vi "DataTranslation.vi"() -> ()   [LabVIEW 2013]
doc: "This vi will take data with multiple DT boxes for an arbitrary number of channels either differentially or single ended, depending upon how you have wired the boxes up."
uses:
  Controls/DT_Cluster.ctl
  Controls/DT_Mode.ctl
  Globals/Meas_global.vi
  <userlib>/LV-Link3/PolySubVIs/DtCreateAinChan.vi
  <userlib>/LV-Link3/PolySubVIs/DtCreateCtrRateChan.vi
  <userlib>/LV-Link3/PolySubVIs/DtOLTimingSetInput.vi
  <userlib>/LV-Link3/PolySubVIs/DtOLStartNormal.vi
  <userlib>/LV-Link3/PolySubVIs/DtOLTriggerDigital.vi
  <userlib>/LV-Link3/PolySubVIs/DtOLReadMultiple2D.vi
panel:
  out "DAQ Error":errorcluster
  out "Array":T1[](array[typedef])
  out "Waveform Graph":dbl[][](graph)
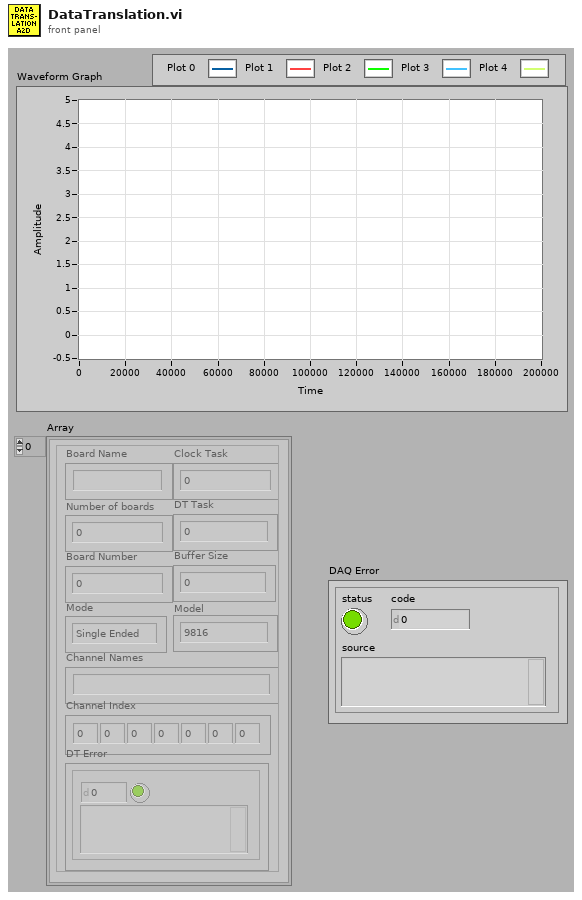
[diagram p1: front panel]
types:
  T1 = typedef "DT_Cluster.ctl" = cluster{"Board Name":string, "Number of boards":u32, "Board Number":u32, "Channel Names":string, "Channel Index":i32[], "DT Task":i32, "DT Error":errorcluster, "Mode":T2, "Buffer Size":u32, "Clock Task":i32, "Model":enum16{"9816", "9836", "9853"}}
  T2 = typedef "DT_Mode.ctl" = enum16{"Single Ended", "Differential"}
  T3 = typedef "Trigger_Mode.ctl" = enum16{"Free Running", "Start on Trigger", "Trigger Every Block", "Trigger Every Sample"}
  T4 = typedef "LDA_Setup.ctl" = cluster{"dimensions":enum16{"1D", "2D"}, "Analogue Freq Multiplier":dbl}
  T5 = enum32{"Internal Clock", "External Clock", "No Timing"}
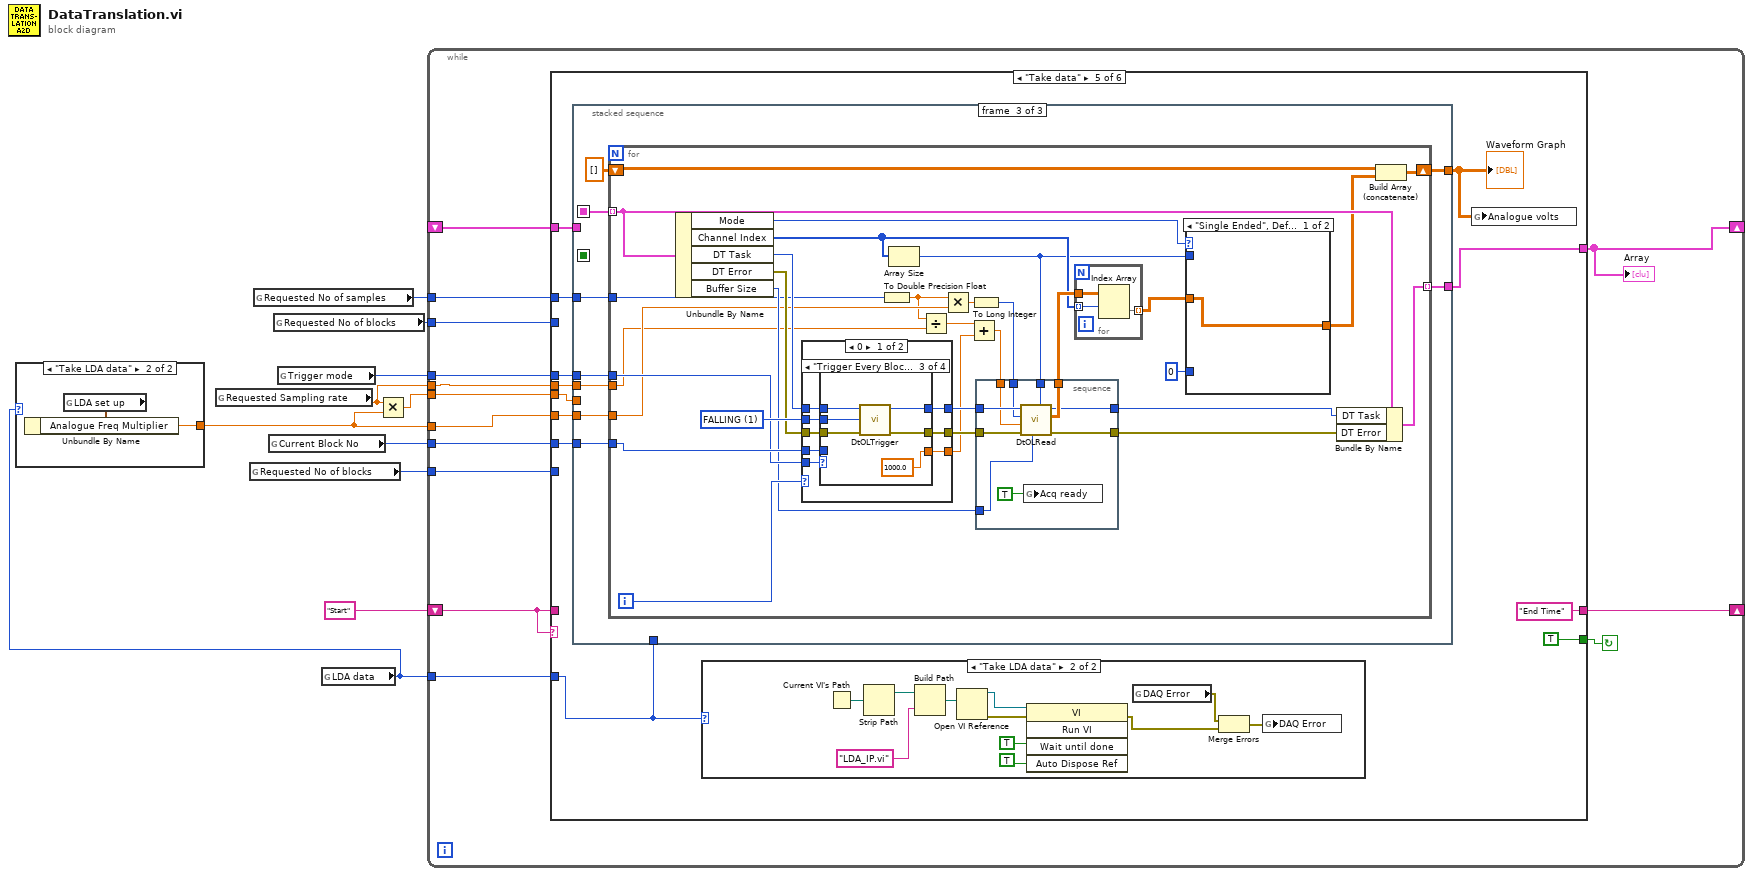
[diagram p0: block diagram]
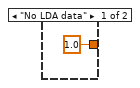
[diagram p2: hidden frame]
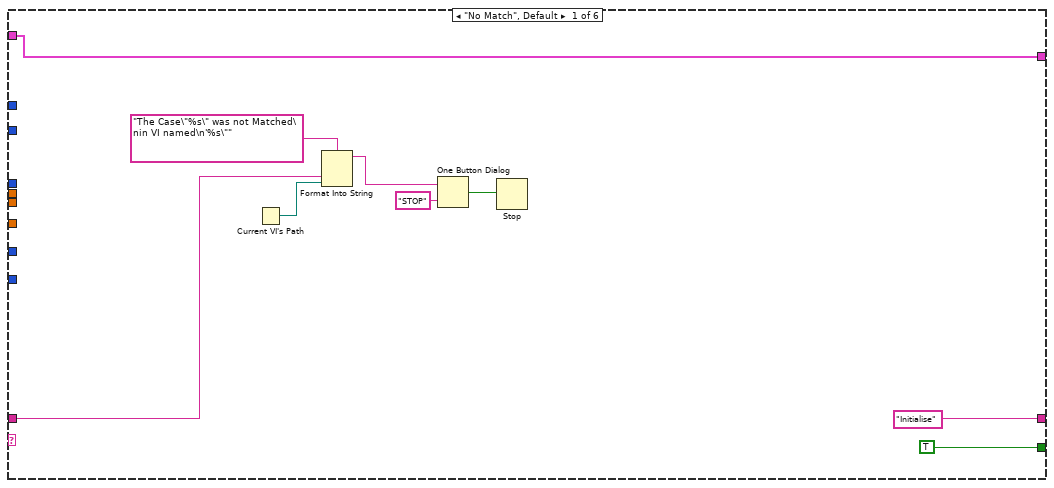
[diagram p3: hidden frame]
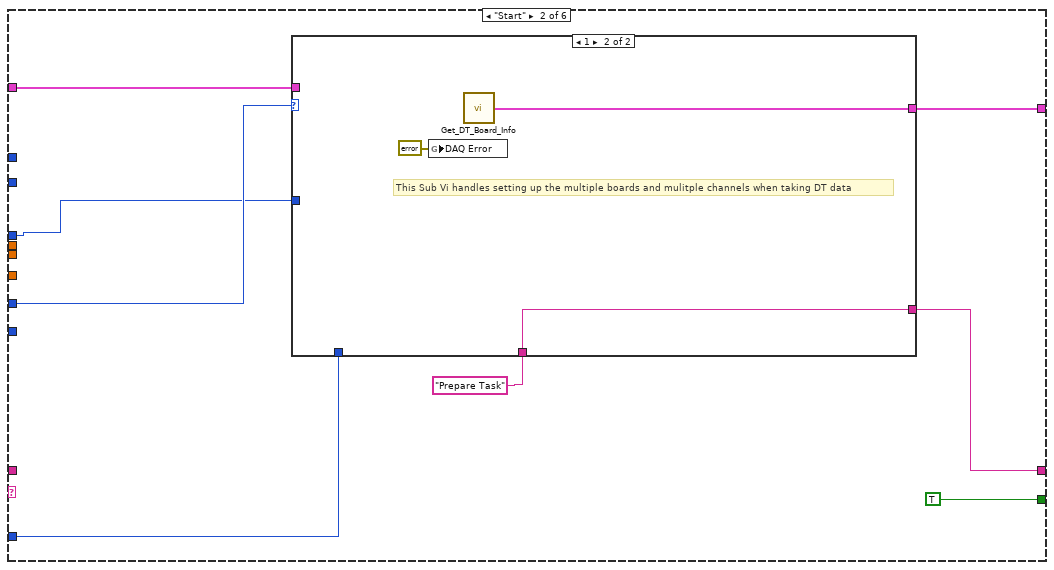
[diagram p4: hidden frame]
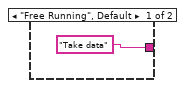
[diagram p6: hidden frame]
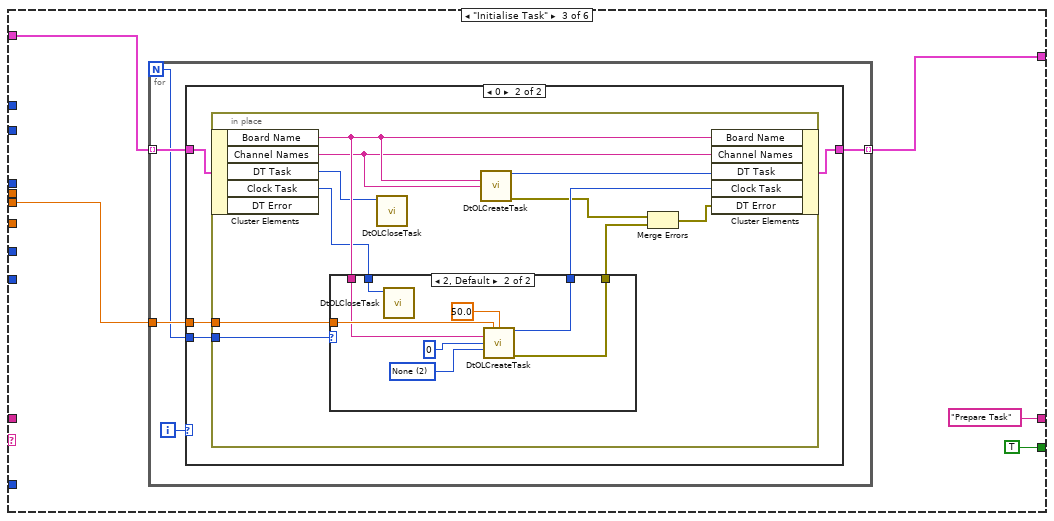
[diagram p8: hidden frame]
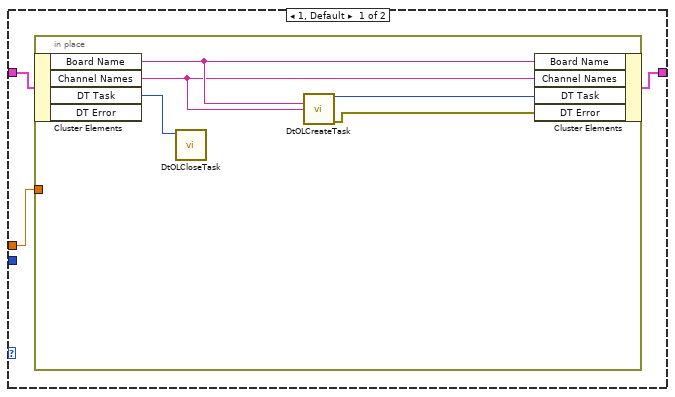
[diagram p9: hidden frame]
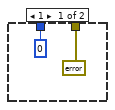
[diagram p10: hidden frame]
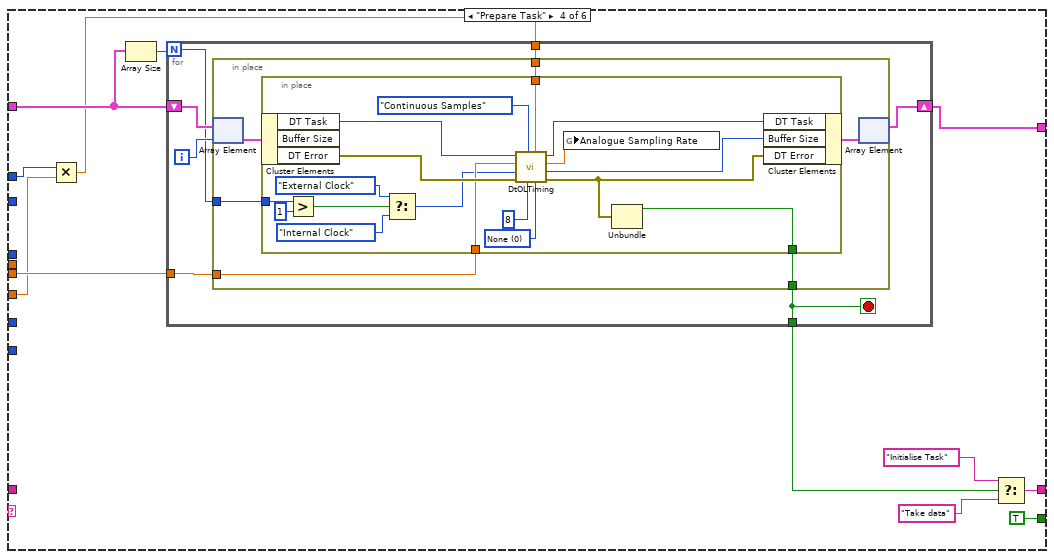
[diagram p11: hidden frame]
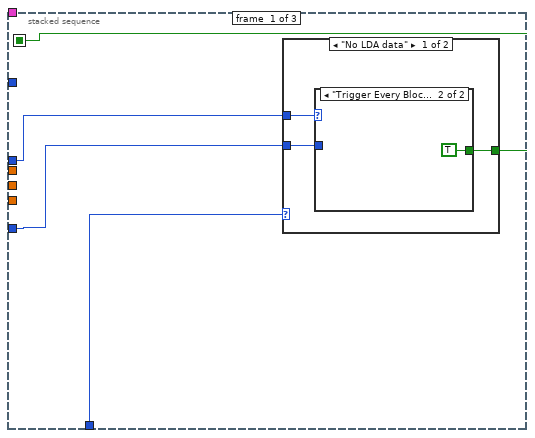
[diagram p13: hidden frame]
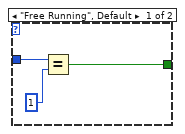
[diagram p14: hidden frame]
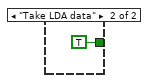
[diagram p15: hidden frame]
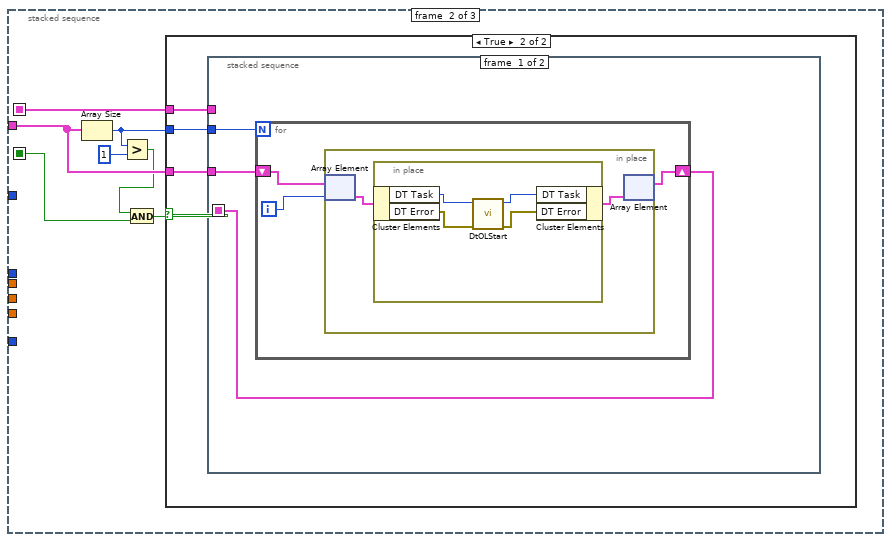
[diagram p16: hidden frame]
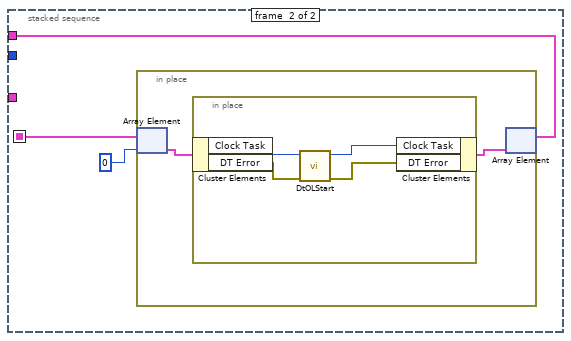
[diagram p18: hidden frame]
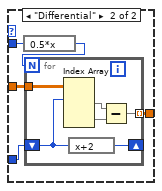
[diagram p19: hidden frame]
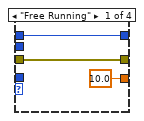
[diagram p20: hidden frame]
diagram:
  n1 = global read "Meas_global.vi" "Requested Sampling rate"() -> (w4:dbl)
  n2 = global read "Meas_global.vi" "Requested No of blocks"() -> (w3:i32)
  n3 = global read "Meas_global.vi" "Requested No of samples"() -> (w9:i32)
  n4 = global read "Meas_global.vi" "Current Block No"() -> (w7:i32)
  n5 = global read "Meas_global.vi" "Requested No of blocks"() -> (w6:i32)
  n6 = global read "Meas_global.vi" "Trigger mode"() -> (w8:T3)
  n7 = global read "Meas_global.vi" "LDA data"() -> (w1:enum16{"No LDA data", "Take LDA data"})
  n8 = case shown="\"Take LDA data\"" w1 {
    tunnel: [1.0 ("Analogue Freq Multiplier") w12] -> w2
    frame "No LDA data" {
    }
    frame "Take LDA data" {
      n9 = global read "Meas_global.vi" "LDA set up"() -> (w13:T4)
      n10 = Unbundle By Name(w13) -> ("Analogue Freq Multiplier"=w12:dbl)
    }
  }
  n11 = Multiply(x=w4, y=w2) -> (x*y=w5:dbl)
  n12 = while {
    shift-left: "Start" -> [w26]
    shift-right: [w27] -> _
    tunnel: w5 -> [w25]
    tunnel: w9 -> [w24]
    tunnel: w7 -> [w23]
    tunnel: w8 -> [w21]
    tunnel: w6 -> [w20]
    shift-right: [w19] -> _
    shift-left: _ -> [w18]
    tunnel: w1 -> [w17]
    tunnel: w2 -> [w16]
    tunnel: w4 -> [w15]
    tunnel: w3 -> [w14]
    stop <- w22 continue-if-true
    n13 = case shown="\"Take data\"" w26 {
      tunnel: ["Initialise" w40 "Prepare Task" w110 "End Time" "" ("f")] -> w27
      tunnel: w26 -> [w32 _ _ _ _ _]
      tunnel: w25 -> [_ _ w61 w106 w145 _]
      tunnel: w24 -> [_ _ _ w104 w155 _]
      tunnel: w23 -> [_ w41 _ _ w153 w319]
      tunnel: [TRUE TRUE TRUE TRUE TRUE FALSE] -> w22
      tunnel: w21 -> [_ w37 _ _ w152 _]
      tunnel: w20 -> [_ _ _ _ _ _]
      tunnel: w18 -> [w28 w42 w59 w105 w151 w323]
      tunnel: [w28 w43 w60 w107 w150 w322] -> w19
      tunnel: w17 -> [_ w38 _ _ w146 _]
      tunnel: w16 -> [_ _ _ w103 w148 _]
      tunnel: w15 -> [_ _ _ _ w147 _]
      tunnel: w14 -> [_ _ _ _ _ w320]
      frame "No Match", Default {
        n14 = Current VI's Path() -> (path=w31:path)
        n15 = Format Into String(format string="The Case\"%s\" was not Matched\nin VI named\n'%s\"" ("Format String"), w32, w31) -> (resulting string=w35:string)  [unwired: 2 in, 1 out]
        n16 = One Button Dialog(message=w35, button name ("OK")="STOP") -> (true=w33:bool)
        n17 = Stop(stop? (T)=w33) -> ()
      }
      frame "Start" {
        n18 = case shown="1" w41 {
          tunnel: [w49 w58] -> w43
          tunnel: w42 -> [w49 _]
          tunnel: [w47 w56] -> w40
          tunnel: "Prepare Task" -> [w46 w56]
          tunnel: w38 -> [w48 _]
          tunnel: w37 -> [w45 _]
          frame 2, Default {
            n19 = case shown="\"No LDA data\"" w48 {
              tunnel: [w52 w55] -> w47
              tunnel: w46 -> [w50 w55]
              tunnel: w45 -> [w51 _]
              frame "No LDA data" {
                n20 = case shown="\"Trigger Every Block\"" w51 {
                  tunnel: ["Take data" w54] -> w52
                  tunnel: w50 -> [_ w54]
                  frame "Free Running", Default {
                  }
                  frame "Trigger Every Block" {
                  }
                }
              }
              frame "Take LDA data" {
              }
            }
          }
          frame 1 {
            # "This Sub Vi handles setting up the multiple boards and mulitple channels when taking DT data"
            n21 = global write "Meas_global.vi" "DAQ Error"(errorcluster {"status"=FALSE, "code"=0, "source"=""} ("DAQ Error")) -> ()
            n22 = call "Get_DT_Board_Info.vi"() -> ("DT Cluster Array"=w58:T1[])  [unwired: 5 in]
          }
        }
      }
      frame "Initialise Task" {
        n23 = for {
          N -> [w64]
          tunnel: w59 -> [w68] mode=indexing
          tunnel: w61 -> [w67]
          tunnel: [w66] -> w60 mode=indexing
          i -> [w65]
          n24 = case shown="0" w65 {
            tunnel: w68 -> [w71 w80]
            tunnel: w67 -> [w70 w79]
            tunnel: [w69 w78] -> w66
            tunnel: w64 -> [_ w77]
            frame 1, Default {
              n25 = in-place {
                in-place-border: w70 -> [_]
                n26 = in-place-cluster #1(w71) -> ("Board Name"=w76:string, "Channel Names"=w73:string, "DT Task"=w72:i32)  [unwired: 1 out]
                n27 = call <userlib>:"DtOLCloseTask.vi"("Task in"=w72) -> ()  [unwired: 10 in, 1 out]
                n28 = call-poly <userlib>:"DtOLCreateTask.vi"("Board Name"=w76, "Channel"=w73) -> ("Task out"=w75:i32, "error out"=w74:errorcluster)  [unwired: 11 in, 1 out]
                n29 = in-place-cluster #1("Board Name"=w76, "Channel Names"=w73, "DT Task"=w75, "DT Error"=w74) -> (w69:T1)
              }
            }
            frame 0 {
              n30 = in-place {
                in-place-border: w79 -> [w91]
                in-place-border: w77 -> [w82]
                n31 = in-place-cluster #2(w80) -> ("Board Name"=w89:string, "Channel Names"=w84:string, "DT Task"=w83:i32, "Clock Task"=w81:i32)  [unwired: 1 out]
                n32 = case shown="2, Default" w82 {
                  tunnel: w91 -> [_ w98]
                  tunnel: [errorcluster {"status"=FALSE, "code"=0, "source"=""} ("error out") w97] -> w90
                  tunnel: w89 -> [_ w96]
                  tunnel: [0 ("Task out") w95] -> w87
                  tunnel: w81 -> [_ w94]
                  frame 1 {
                  }
                  frame 2, Default {
                    w101 = 2 items=["LowLevel", "HighLevel", "None"] ("Gate Type")
                    n33 = call <userlib>:"DtOLCloseTask.vi"("Task in"=w94) -> ()  [unwired: 10 in, 1 out]
                    n34 = call-poly <userlib>:"DtOLCreateTask.vi"("Requested\nFrequency (Hz)"=w98, "Duty Cycle"=50.0, "Board Name"=w96, "Counter Num"=u32 0, "Gate Type"=w101) -> ("Task out"=w95:i32, "error out"=w97:errorcluster)  [unwired: 8 in, 1 out]
                  }
                }
                n35 = call <userlib>:"DtOLCloseTask.vi"("Task in"=w83) -> ()  [unwired: 10 in, 1 out]
                n36 = call-poly <userlib>:"DtOLCreateTask.vi"("Board Name"=w89, "Channel"=w84) -> ("Task out"=w88:i32, "error out"=w86:errorcluster)  [unwired: 11 in, 1 out]
                n37 = Merge Errors(w86, w90) -> (w85:errorcluster)
                n38 = in-place-cluster #2("Board Name"=w89, "Channel Names"=w84, "DT Task"=w88, "Clock Task"=w87, "DT Error"=w85) -> (w78:T1)
              }
            }
          }
        }
      }
      frame "Prepare Task" {
        n39 = Multiply(x=w104, y=w103) -> (x*y=w102:dbl)
        n40 = Array Size(array=w105) -> (size(s)=w109:i32)
        n41 = for {
          N: w109 -> [w114]
          shift-right: [w117] -> w107
          shift-left: w105 -> [w119]
          tunnel: [w120] -> w108
          tunnel: w106 -> [w116]
          tunnel: w102 -> [w115]
          i -> [w118]
          stop <- w120 stop-if-true
          n42 = in-place {
            in-place-border: [w126] -> w120
            in-place-border: w116 -> [w123]
            in-place-border: w115 -> [w122]
            in-place-border: w114 -> [w121]
            n43 = in-place-array #3(w119, w118) -> (w125:T1)
            n44 = in-place {
              in-place-border: [w138] -> w126
              in-place-border: w123 -> [w137]
              in-place-border: w122 -> [w136]
              in-place-border: w121 -> [w135]
              w128 = 0 items=["None", "Master", "Slave"] ("Sync Mode")
              n45 = in-place-cluster #4(w125) -> ("DT Task"=w143:i32, "DT Error"=w142:errorcluster)  [unwired: 1 out]
              n46 = Greater?(x=w135, y=1) -> (0:w133:bool)
              n47 = Select(t=T5."External Clock" ("Timing"), s=w133, f=T5."Internal Clock" ("Timing")) -> (s? t:f=w130:T5)
              n48 = call-poly <userlib>:"DtOLTiming.vi"("Sync Mode"=w128, "Samples Per Channel"=w136, "Num Buffers"=u32 8, "Sample Mode"=enum16{"Finite Samples", "Continuous Samples"}."Continuous Samples", "error in (no error)"=w142, "Timing"=w130, "Sample Freq (Hz)"=w137, "Task in"=w143) -> ("error out"=w139:errorcluster, "Buffer Size"=w141:u32, "Actual Sample Freq"=w144:dbl, "Task out"=w140:i32)
              n49 = global write "Meas_global.vi" "Analogue Sampling Rate"(w144) -> ()
              n50 = Unbundle(w139) -> ("status"=w138:bool)  [unwired: 2 out]
              n51 = in-place-cluster #4("DT Task"=w140, "Buffer Size"=w141, "DT Error"=w139) -> (w124:T1)
            }
            n52 = in-place-array #3(w124) -> (w117:T1[])  [unwired: 1 out]
          }
        }
        n53 = Select(t="Initialise Task", s=w108, f="Take data") -> (s? t:f=w110:string)
      }
      frame "Take data" {
        n54 = stacked-sequence {
          seq-local: [_ w186 _] -> [_ _ w212]
          seq-local: [w169 _ _] -> [_ w181 _]
          tunnel: w155 -> [_ _ w220]
          tunnel: w153 -> [w170 _ w219]
          tunnel: w152 -> [w168 _ w218]
          tunnel: w151 -> [_ w185 _]
          tunnel: [_ _ w217] -> w150
          tunnel: [_ _ w215] -> w149
          tunnel: w148 -> [_ _ w214]
          tunnel: w147 -> [_ _ w213]
          tunnel: w146 -> [w171 _ _]
          tunnel: w145 -> [_ _ _]
          frame #0 {
            n55 = case shown="\"No LDA data\"" w171 {
              tunnel: w170 -> [w174 _]
              tunnel: [w173 TRUE] -> w169
              tunnel: w168 -> [w172 _]
              frame "No LDA data" {
                n56 = case shown="\"Trigger Every Block\"" w172 {
                  tunnel: w174 -> [w177 _]
                  tunnel: [w175 TRUE] -> w173
                  frame "Free Running", Default {
                    n57 = Equal?(x=w177, y=1) -> (x = y?=w175:bool)
                  }
                  frame "Trigger Every Block" {
                  }
                }
              }
              frame "Take LDA data" {
              }
            }
          }
          frame #1 {
            n58 = Array Size(array=w185) -> (size(s)=w184:i32)
            n59 = Greater?(x=w184, y=1) -> (0:w182:bool)
            n60 = And(x=w182, y=w181) -> (x .and. y?=w180:bool)
            n61 = case shown="True" w180 {
              tunnel: [w187 w190] -> w186
              tunnel: w185 -> [w187 w189]
              tunnel: w184 -> [_ w188]
              frame False {
              }
              frame True {
                n62 = stacked-sequence {
                  seq-local: [w191 _] -> [_ w204]
                  tunnel: [_ w203] -> w190
                  tunnel: w189 -> [w193 _]
                  tunnel: w188 -> [w192 _]
                  frame #0 {
                    n63 = for {
                      N: w192 -> [_]
                      shift-right: [w194] -> w191
                      shift-left: w193 -> [w195]
                      i -> [w196]
                      n64 = in-place {
                        n65 = in-place-array #5(w195, w196) -> (w198:T1)
                        n66 = in-place {
                          n67 = in-place-cluster #6(w198) -> ("DT Task"=w202:i32, "DT Error"=w201:errorcluster)
                          n68 = call-poly <userlib>:"DtOLStart.vi"("error in (no error)"=w201, "Task in"=w202) -> ("error out"=w200:errorcluster, "Task out"=w199:i32)  [unwired: 8 in]
                          n69 = in-place-cluster #6("DT Task"=w199, "DT Error"=w200) -> (w197:T1)
                        }
                        n70 = in-place-array #5(w197) -> (w194:T1[])  [unwired: 1 out]
                      }
                    }
                  }
                  frame #1 {
                    n71 = in-place {
                      n72 = in-place-array #7(w204, 0) -> (w207:T1)
                      n73 = in-place {
                        n74 = in-place-cluster #8(w207) -> ("Clock Task"=w210:i32, "DT Error"=w211:errorcluster)
                        n75 = call-poly <userlib>:"DtOLStart.vi"("error in (no error)"=w211, "Task in"=w210) -> ("error out"=w208:errorcluster, "Task out"=w209:i32)  [unwired: 8 in]
                        n76 = in-place-cluster #8("Clock Task"=w209, "DT Error"=w208) -> (w206:T1)
                      }
                      n77 = in-place-array #7(w206) -> (w203:T1[])  [unwired: 1 out]
                    }
                  }
                }
              }
            }
          }
          frame #2 {
            n78 = for {
              tunnel: w220 -> [w230]
              tunnel: w219 -> [w249]
              tunnel: w218 -> [w248]
              tunnel: w212 -> [w244] mode=indexing
              tunnel: [w243] -> w217 mode=indexing
              shift-right: [w240] -> w215
              shift-left: dbl[][] [] -> [w239]
              tunnel: w214 -> [w229]
              tunnel: w213 -> [w227]
              i -> [w237]
              w250 = 1 items=["RISING", "FALLING"] ("External Trigger Polarity")
              n79 = Unbundle By Name(w244) -> ("Mode"=w234:T2, "Channel Index"=w241:i32[], "DT Task"=w247:i32, "DT Error"=w246:errorcluster, "Buffer Size"=w232:u32)
              n80 = case shown="0" w237 {
                tunnel: [w281 w312] -> w251
                tunnel: w250 -> [w280 _]
                tunnel: w249 -> [w279 _]
                tunnel: w248 -> [w278 _]
                tunnel: w247 -> [w277 w312]
                tunnel: w246 -> [w276 w311]
                tunnel: [w275 w311] -> w245
                tunnel: [w274 10.0 ("x")] -> w224
                frame 0 {
                  n81 = case shown="\"Trigger Every Block\"" w278 {
                    tunnel: [w284 w289 w304 w309] -> w281
                    tunnel: w277 -> [w284 w290 w306 w309]
                    tunnel: w279 -> [_ w291 _ _]
                    tunnel: w280 -> [_ w288 w305 _]
                    tunnel: w276 -> [w283 w287 w303 w308]
                    tunnel: [w283 w286 w302 w308] -> w275
                    tunnel: [10.0 ("x") w285 1000.0 ("x") 1000.0 ("x")] -> w274
                    frame "Free Running" {
                    }
                    frame "Start on Trigger" {
                      n82 = case shown="1" w291 {
                        tunnel: w290 -> [w297 w300]
                        tunnel: w287 -> [w296 w299]
                        tunnel: [w294 w300] -> w289
                        tunnel: [w295 w299] -> w286
                        tunnel: w288 -> [w293 _]
                        tunnel: [1000.0 ("x") 10.0 ("x")] -> w285
                        frame 1 {
                          n83 = call-poly <userlib>:"DtOLTrigger.vi"("error in (no error)"=w296, "External Trigger Polarity"=w293, "Task in"=w297) -> ("error out"=w295:errorcluster, "Task out"=w294:i32)  [unwired: 7 in]
                        }
                        frame 2, Default {
                        }
                      }
                    }
                    frame "Trigger Every Block" {
                      n84 = call-poly <userlib>:"DtOLTrigger.vi"("error in (no error)"=w303, "External Trigger Polarity"=w305, "Task in"=w306) -> ("error out"=w302:errorcluster, "Task out"=w304:i32)  [unwired: 7 in]
                    }
                    frame "Trigger Every Sample" {
                    }
                  }
                }
                frame 1, Default {
                }
              }
              n85 = To Double Precision Float(number=w230) -> (double precision float=w222:dbl)
              n86 = Array Size(array=w241) -> (size(s)=w223:i32)
              n87 = Divide(x=w222, y=w227) -> (x/y=w225:dbl)
              n88 = Multiply(x=w222, y=w229) -> (x*y=w228:dbl)
              n89 = Add(x=w225, y=w224) -> (x+y=w238:dbl)
              n90 = To Long Integer(number=w228) -> (32bit integer=w221:i32)
              n91 = stacked-sequence {
                tunnel: w251 -> [w261]
                tunnel: w245 -> [w260]
                tunnel: [w259] -> w242
                tunnel: w238 -> [w258]
                tunnel: [w257] -> w236
                tunnel: w232 -> [w253]
                tunnel: [w256] -> w231
                tunnel: w221 -> [w255]
                tunnel: w223 -> [w254]
                frame #0 {
                  n92 = call-poly <userlib>:"DtOLRead.vi"("Number Chan to Read"=w254, "Buffer size"=w253, "error in (no error)"=w260, "Timeout"=w258, "Samples Per Channel"=w255, "Task in"=w261) -> ("error out"=w256:errorcluster, "2D Data out"=w259:dbl[][], "Task out"=w257:i32)  [unwired: 1 in, 2 out]
                  n93 = global write "Meas_global.vi" "Acq ready"(TRUE ("Acq ready")) -> ()
                }
              }
              n94 = for {
                tunnel: w241 -> [w315] mode=indexing
                tunnel: w242 -> [w314]
                tunnel: [w313] -> w226 mode=indexing
                n95 = Index Array(array=w314, index (row)=w315) -> (element=w313:dbl[])  [unwired: 1 in]
              }
              n96 = case shown="\"Single Ended\", Default" w234 {
                tunnel: w226 -> [w262 w267]
                tunnel: [w262 w266] -> w235
                tunnel: 0 ("size(s)") -> [_ w265]
                tunnel: w223 -> [_ w264]
                frame "Single Ended", Default {
                }
                frame "Differential" {
                  n97 = expression code="0.5*x"(w264) -> (w263:i32)
                  n98 = for {
                    N: w263 -> [_]
                    tunnel: w267 -> [w273]
                    shift-right: [w272] -> _
                    shift-left: w265 -> [w271]
                    tunnel: [w269] -> w266 mode=indexing
                    n99 = Index Array(array=w273, index (row) #1=w271) -> (element #1=w268:dbl[], element #2=w270:dbl[])  [unwired: 3 in]
                    n100 = expression code="x+2"(w271) -> (w272:i32)
                    n101 = Subtract(x=w268, y=w270) -> (x-y=w269:dbl[])
                  }
                }
              }
              n102 = Bundle By Name(cluster=w244, "DT Task"=w236, "DT Error"=w231) -> (w243:T1)
              n103 = Build Array (concatenate)(w239, w235) -> (w240:dbl[][])
            }
          }
        }
        "Waveform Graph" <- w149
        n104 = case shown="\"Take LDA data\"" w146 {
          frame "No LDA data", Default {
          }
          frame "Take LDA data" {
            n105 = Current VI's Path() -> (path=w161:path)
            n106 = Strip Path(path=w161) -> (stripped path=w157:path)  [unwired: 1 out]
            n107 = Build Path(base path=w157, name or relative path="LDA_IP.vi") -> (appended path=w162:path)
            n108 = Open VI Reference(vi path=w162) -> (vi reference=w165:refnum<vi>, error out=w166:errorcluster)  [unwired: 5 in]
            n109 = invoke class="VI" method="Run VI"(reference=w165, error in=w166, "Wait until done"=TRUE ("Wait Until Done"), "Auto Dispose Ref"=TRUE ("Wait until done")) -> (error out=w159:errorcluster)  [unwired: 1 in, 4 out]
            n110 = global read "Meas_global.vi" "DAQ Error"() -> (w160:errorcluster)
            n111 = Merge Errors(w160, w159) -> (w158:errorcluster)
            n112 = global write "Meas_global.vi" "DAQ Error"(w158) -> ()
          }
        }
        n113 = global write "Meas_global.vi" "Analogue volts"(w149) -> ()
      }
      frame "End Time" {
        n114 = Equal?(x=w319, y=w320) -> (x = y?=w317:bool)
        n115 = case shown="True" w317 {
          tunnel: w323 -> [w326 w328]
          tunnel: [w326 w327] -> w322
          frame False {
          }
          frame True {
            n116 = for {
              N -> [w329]
              tunnel: w328 -> [w332] mode=indexing
              tunnel: [w331] -> w327 mode=indexing
              i -> [w330]
              n117 = case shown="0" w330 {
                tunnel: w332 -> [w334 w341]
                tunnel: [w333 w340] -> w331
                tunnel: w329 -> [_ w339]
                frame 1, Default {
                  n118 = in-place {
                    n119 = in-place-cluster #9(w334) -> ("DT Task"=w338:i32, "DT Error"=w337:errorcluster)
                    n120 = call <userlib>:"DtOLCloseTask.vi"("Error in"=w337, "Task in"=w338) -> ("Error Out"=w336:errorcluster)  [unwired: 9 in]
                    n121 = in-place-cluster #9("DT Task"=0, "DT Error"=w336) -> (w333:T1)
                  }
                }
                frame 0 {
                  n122 = in-place {
                    in-place-border: w339 -> [w342]
                    n123 = in-place-cluster #10(w341) -> ("DT Task"=w348:i32, "DT Error"=w347:errorcluster, "Clock Task"=w345:i32)
                    n124 = case shown="2, Default" w342 {
                      tunnel: [errorcluster {"status"=FALSE, "code"=0, "source"=""} ("Error Out") w353] -> w350
                      tunnel: w345 -> [_ w352]
                      frame 1 {
                      }
                      frame 2, Default {
                        n125 = call <userlib>:"DtOLCloseTask.vi"("Task in"=w352) -> ("Error Out"=w353:errorcluster)  [unwired: 10 in]
                      }
                    }
                    n126 = call <userlib>:"DtOLCloseTask.vi"("Error in"=w347, "Task in"=w348) -> ("Error Out"=w346:errorcluster)  [unwired: 9 in]
                    n127 = Merge Errors(w346, w350) -> (w349:errorcluster)
                    n128 = in-place-cluster #10("DT Task"=0, "DT Error"=w349, "Clock Task"=0) -> (w340:T1)
                  }
                }
              }
            }
          }
        }
        n129 = global read "Meas_global.vi" "DAQ Error"() -> (w318:errorcluster)
        n130 = for {
          tunnel: w322 -> [w357] mode=indexing
          shift-right: [w354] -> w321
          shift-left: w318 -> [w355]
          n131 = Unbundle By Name(w357) -> ("DT Error"=w356:errorcluster)
          n132 = Merge Errors(w355, w356) -> (w354:errorcluster)
        }
        "DAQ Error" <- w321
        n133 = global write "Meas_global.vi" "DAQ Error"(w321) -> ()
        n134 = global write "Meas_global.vi" "Acq ready"(FALSE ("Acq ready")) -> ()
      }
    }
    "Array" <- w19
  }
